vi "MecaDrivePoseEst_New.vi"(5 "gyroAngle":T5={"VALUE"=0.0, "COS"=1.0, "SIN"=0.0} {"SIN" format="%13.4f"; "COS" format="%13.4f"; "VALUE" format="%13.4f"}, 6 "MecanumKinematics":T1={"FrontLeft"={"X"=0.0, "Y"=0.0}, "FrontRight"={"X"=0.0, "Y"=0.0}, "RearLeft"={"X"=0.0, "Y"=0.0}, "RearRight"={"X"=0.0, "Y"=0.0}, "InverseKinematics"=[[0.0, 1.0, -1.0, 0.0], [0.0, 1.0, 1.0, 0.0], [0.0, 1.0, 1.0, 0.0], [0.0, 1.0, -1.0, 0.0]], "ForwardKinematics"=[[0.0, 1.0, -1.0, 0.0], [0.0, 1.0, 1.0, 0.0], [0.0, 1.0, 1.0, 0.0], [0.0, 1.0, -1.0, 0.0]], "PrevCoR"={"X"=0.0, "Y"=0.0}} {"PrevCoR"."Y" format="%14.3f"; "PrevCoR"."X" format="%14.3f"; "RearRight"."Y" format="%14.3f"; "RearRight"."X" format="%14.3f"; "RearLeft"."Y" format="%14.3f"; "RearLeft"."X" format="%14.3f"; "FrontRight"."Y" format="%14.3f"; "FrontRight"."X" format="%14.3f"; "FrontLeft"."Y" format="%14.3f"; "FrontLeft"."X" format="%14.3f"}, 7 "InitialPose":T4={"TRANSLATION"={"X"=0.0, "Y"=0.0}, "ROTATION"={"VALUE"=0.0, "COS"=1.0, "SIN"=0.0}} {"ROTATION"."SIN" format="%13.4f"; "ROTATION"."COS" format="%13.4f"; "ROTATION"."VALUE" format="%13.4f"; "TRANSLATION"."Y" format="%14.3f"; "TRANSLATION"."X" format="%14.3f"}, 8 "dt_Seconds":dbl=0.02, 9 "VisionMeasurementStdDevs":T3=[[0.0], [0.0], [0.0]], 10 "LocalMeasurementStdDevs":T3=[[0.0]], 11 "StateStdDevs":T3=[[0.0], [0.0], [0.0]]) -> (0 "Error":errorcluster, 3 "MecaDrivePoseEstimate":T6={"M_VisionContR"=[], "m_nominal_dT"=0.0, "m_PrevTime_Sec"=0.0, "m_GyroOffset"={"VALUE"=0.0, "COS"=1.0, "SIN"=0.0}, "m_PrevAngle"={"VALUE"=0.0, "COS"=1.0, "SIN"=0.0}, "m_Observer"={"m_P"=[], "m_xHat"=[], "States"=0, "Outputs"=0, "m_ContR"=[], "m_ContQ"=[], "m_SigmasF"=[], "m_dT_Sec"=0.0, "MERWE_SCALED_SIGMA_PTS"={"m_Wm"=[], "States"=0, "Alpha"=0.0, "m_Wc"=[], "Kappa"=0}, "meanFuncX"=refnum, "meanFuncY"=refnum, "residualFuncX"=refnum, "residualFuncY"=refnum, "addFuncX"=refnum, "addFuncXExtra"=variant, "residualFuncYExtra"=variant, "residualFuncXExtra"=variant, "MeanFuncYExtra"=variant, "MeanFuncXExtra"=variant, "Inputs"=0}, "m_kinematics"={"FrontLeft"={"X"=0.0, "Y"=0.0}, "FrontRight"={"X"=0.0, "Y"=0.0}, "RearLeft"={"X"=0.0, "Y"=0.0}, "RearRight"={"X"=0.0, "Y"=0.0}, "InverseKinematics"=[[0.0, 1.0, -1.0, 0.0], [0.0, 1.0, 1.0, 0.0], [0.0, 1.0, 1.0, 0.0], [0.0, 1.0, -1.0, 0.0]], "ForwardKinematics"=[[0.0, 1.0, -1.0, 0.0], [0.0, 1.0, 1.0, 0.0], [0.0, 1.0, 1.0, 0.0], [0.0, 1.0, -1.0, 0.0]], "PrevCoR"={"X"=0.0, "Y"=0.0}}, "Pose_Buffer"={"TimeStamps"=[], "Pose"=[], "Min_TimeStamp"=0.0, "Max_TimeStamp"=0.0, "ItemCount"=0, "MaxBufferTime"=0.0}} {"Pose_Buffer"."Pose"."ROTATION"."SIN" format="%13.4f"; "Pose_Buffer"."Pose"."ROTATION"."COS" format="%13.4f"; "Pose_Buffer"."Pose"."ROTATION"."VALUE" format="%13.4f"; "Pose_Buffer"."Pose"."TRANSLATION"."Y" format="%14.3f"; "Pose_Buffer"."Pose"."TRANSLATION"."X" format="%14.3f"; "m_kinematics"."PrevCoR"."Y" format="%14.3f"; "m_kinematics"."PrevCoR"."X" format="%14.3f"; "m_kinematics"."RearRight"."Y" format="%14.3f"; "m_kinematics"."RearRight"."X" format="%14.3f"; "m_kinematics"."RearLeft"."Y" format="%14.3f"; "m_kinematics"."RearLeft"."X" format="%14.3f"; "m_kinematics"."FrontRight"."Y" format="%14.3f"; "m_kinematics"."FrontRight"."X" format="%14.3f"; "m_kinematics"."FrontLeft"."Y" format="%14.3f"; "m_kinematics"."FrontLeft"."X" format="%14.3f"; "m_PrevAngle"."SIN" format="%13.4f"; "m_PrevAngle"."COS" format="%13.4f"; "m_PrevAngle"."VALUE" format="%13.4f"; "m_GyroOffset"."SIN" format="%13.4f"; "m_GyroOffset"."COS" format="%13.4f"; "m_GyroOffset"."VALUE" format="%13.4f"})   [LabVIEW 2019, in "Trajectory_Library.lvlib"]
doc: "Constructs a SwerveDrivePoseEstimator.\n\nThis class wraps an UnscentedKalmanFilter Unscented Kalman Filter to fuse latency-compensated vision measurements with swerve drive encoder velocity measurements. It will correct for noisy measurements and encoder drift. It is intended to be an easy but more accurate drop-in for SwerveDriveOdometry.\n \nSwerveDrivePoseEstimator_update should be called every robot loop. If your loops are faster or slower than the default of 0.02s, then you should change the nominal delta time using the calling parameter. \n \nSwerveDrivePoseEstimator_addVisionMeasurement can be called as infrequently as you want; if you never call it, then this class will behave mostly like regular encoder odometry.\n \nThe state-space system used internally has the following states (x), inputs (u), and outputs\n(y):\n \n x = [x, y, theta]? \n in the field coordinate system containing x position, \n y position, and heading.\n \n u = [v_l, v_r, dtheta]? \n containing left wheel velocity, right wheel velocity, \n and change in gyro heading.\n \n y = [x, y, theta]?\n from vision containing x position, y position, and\n heading; or <strong> y = [theta]? </strong> containing \n gyro heading.\n \n \nInputs:\n - gyroAngle -- The current gyro angle.\n - initialPoseMeters -- The starting pose estimate.\n - stateStdDevs -- Standard deviations of model states. Increase these numbers \n to trust your model's state estimates less. This matrix is in the form \n [x, y, theta]?, with units in meters and radians.\n - localMeasurementStdDevs -- Standard deviations of the encoder and gyro \n measurements. Increase these numbers to trust sensor readings from encoders \n and gyros less. This matrix is in the form [theta], with units in radians.\n - visionMeasurementStdDevs -- Standard deviations of the vision measurements. \n Increase these numbers to trust global measurements from vision less. \n This matrix is in the form [x, y,theta]?, with units in meters and radians.\n - nominalDtSeconds -- The time in seconds between each robot loop.\n - SwerveKinematics -- A correctly-configured kinematics object for your drivetrain.\n\n\nOutputs:\n - outSwevePoseEst -- Updated data cluster \n - Error -- If TRUE, an error occured."
uses:
  Trajectory_Library.lvlib
  MECA_DRIVE_POSE_EST.ctl
  <vilib>/Analysis/Matrix/Datatypes/RealMatrix.ctl
  ROTATION2D.ctl
  UNSCENTED_KALMAN_FILTER.ctl
  MERWE_SCALED_SIGMA_PTS.ctl
  CALLBACK_FUNC_TYPE.ctl
  MECA_DRIVE_KINEMATICS.ctl
  TRANSLATION2D.ctl
  TIME_INTERPOLATABLE_POSE.ctl
  POSE2D.ctl
  MatBuilder_Create.vi
  VecBuilder_3x1Fill.vi
  Pose2d_getXYAngle.vi
  Rotation2d_UnaryMinus.vi
  Rotation2d_RotateBy.vi
  Rotation2d_CreateAngle.vi
  Rotation2d_CreateXY.vi
  Util_CalcDist.vi
  <vilib>/Analysis/Matrix/NI_Matrix.lvlib
panel:
  in  "RightDistance_M":dbl
  in  "LeftDistance_M":dbl
  # "<3,1>"
  # "<1, 1>"
  # "<3, 1>"
  # "<3, 3>"
  # "State Estimate <Statess,1>"
  # "<States, States>"
  # "<States, ?>"
  # "<Statess,  States>"
  # "<Outputs, Outputs>"
  # "<?, 1>"
  # "<?, 1>"
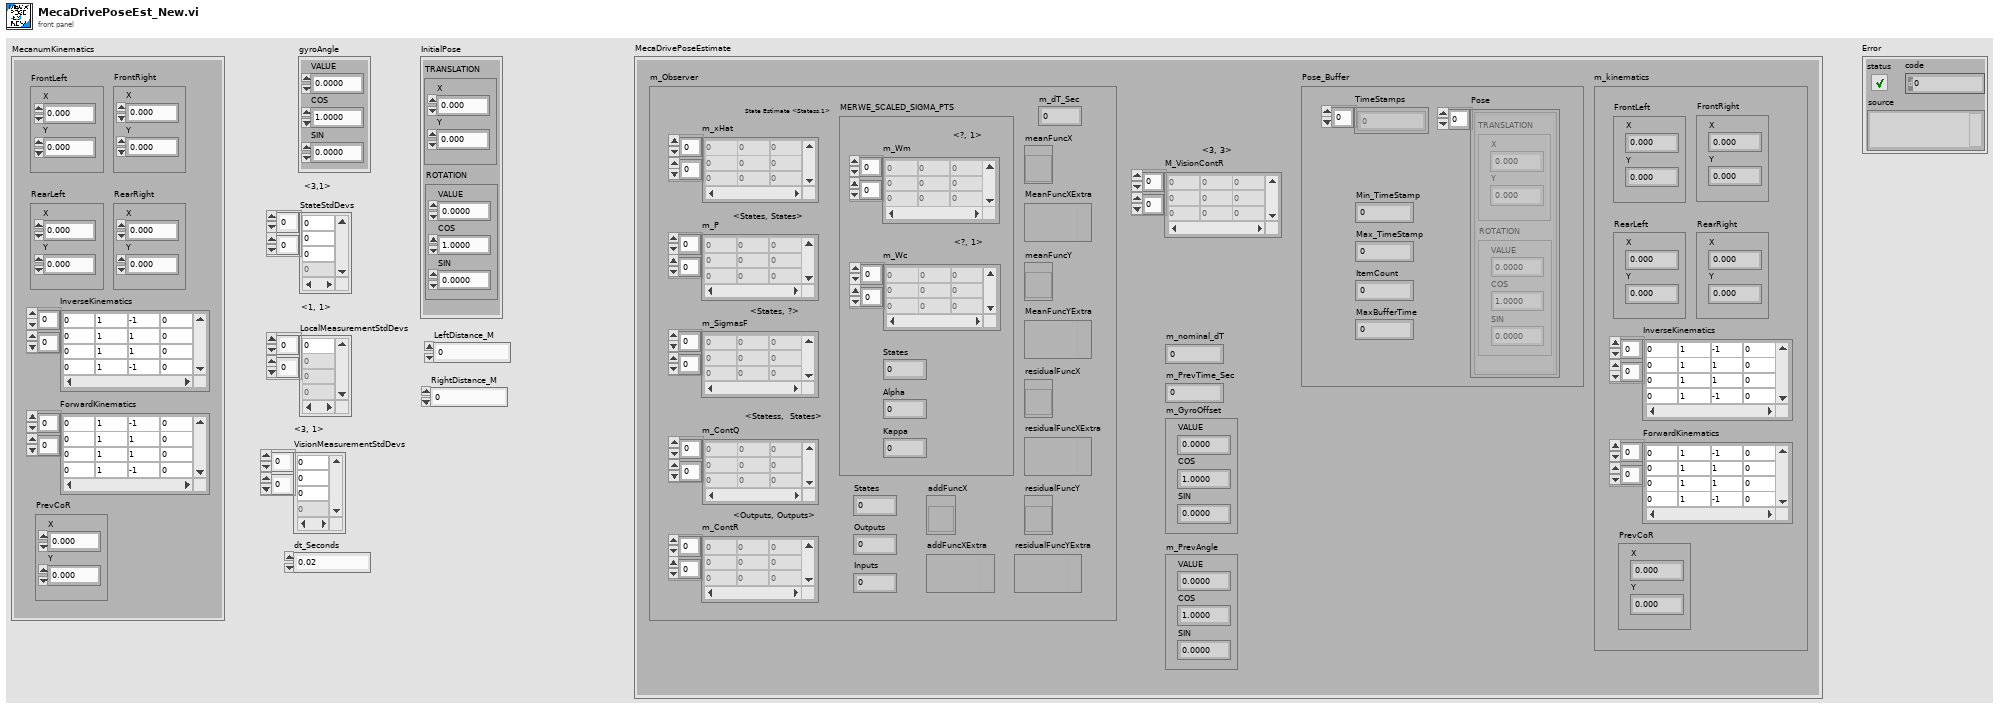
[diagram p1: front panel]
types:
  T1 = typedef "Trajectory_Library.lvlib/MECA_DRIVE_KINEMATICS.ctl" = cluster{"FrontLeft":T2, "FrontRight":T2, "RearLeft":T2, "RearRight":T2, "InverseKinematics":T3, "ForwardKinematics":T3, "PrevCoR":T2}
  T2 = typedef "Trajectory_Library.lvlib/TRANSLATION2D.ctl" = cluster{"X":dbl, "Y":dbl}
  T3 = typedef "NI_Matrix.lvlib/RealMatrix.ctl" = dbl[][]
  T4 = typedef "Trajectory_Library.lvlib/POSE2D.ctl" = cluster{"TRANSLATION":T2, "ROTATION":T5}
  T5 = typedef "Trajectory_Library.lvlib/ROTATION2D.ctl" = cluster{"VALUE":dbl, "COS":dbl, "SIN":dbl}
  T6 = typedef "Trajectory_Library.lvlib/MECA_DRIVE_POSE_EST.ctl" = cluster{"M_VisionContR":T3, "m_nominal_dT":dbl, "m_PrevTime_Sec":dbl, "m_GyroOffset":T5, "m_PrevAngle":T5, "m_Observer":T7, "m_kinematics":T1, "Pose_Buffer":T10}
  T7 = typedef "Trajectory_Library.lvlib/UNSCENTED_KALMAN_FILTER.ctl" = cluster{"m_P":T3, "m_xHat":T3, "States":i32, "Outputs":i32, "m_ContR":T3, "m_ContQ":T3, "m_SigmasF":T3, "m_dT_Sec":dbl, "MERWE_SCALED_SIGMA_PTS":T8, "meanFuncX":T9, "meanFuncY":T9, "residualFuncX":T9, "residualFuncY":T9, "addFuncX":T9, "addFuncXExtra":variant, "residualFuncYExtra":variant, "residualFuncXExtra":variant, "MeanFuncYExtra":variant, "MeanFuncXExtra":variant, "Inputs":i32}
  T8 = typedef "Trajectory_Library.lvlib/MERWE_SCALED_SIGMA_PTS.ctl" = cluster{"m_Wm":T3, "States":i32, "Alpha":dbl, "m_Wc":T3, "Kappa":i32}
  T9 = typedef "Trajectory_Library.lvlib/CALLBACK_FUNC_TYPE.ctl" = refnum<vi>
  T10 = typedef "Trajectory_Library.lvlib/TIME_INTERPOLATABLE_POSE.ctl" = cluster{"TimeStamps":dbl[], "Pose":T4[], "Min_TimeStamp":dbl, "Max_TimeStamp":dbl, "ItemCount":i32, "MaxBufferTime":dbl}
  T11 = typedef "Trajectory_Library.lvlib/UNSCENTED_KALMAN_NEW_FUNC_GROUP.ctl" = cluster{"meanFuncX":T9, "meanFuncY":T9, "residualFuncX":T9, "residualFuncY":T9, "addFuncX":T9, "MeanFuncXExtra":variant, "MeanFuncYExtra":variant, "residualFuncXExtra":variant, "residualFuncYExtra":variant, "addFuncXExtra":variant}
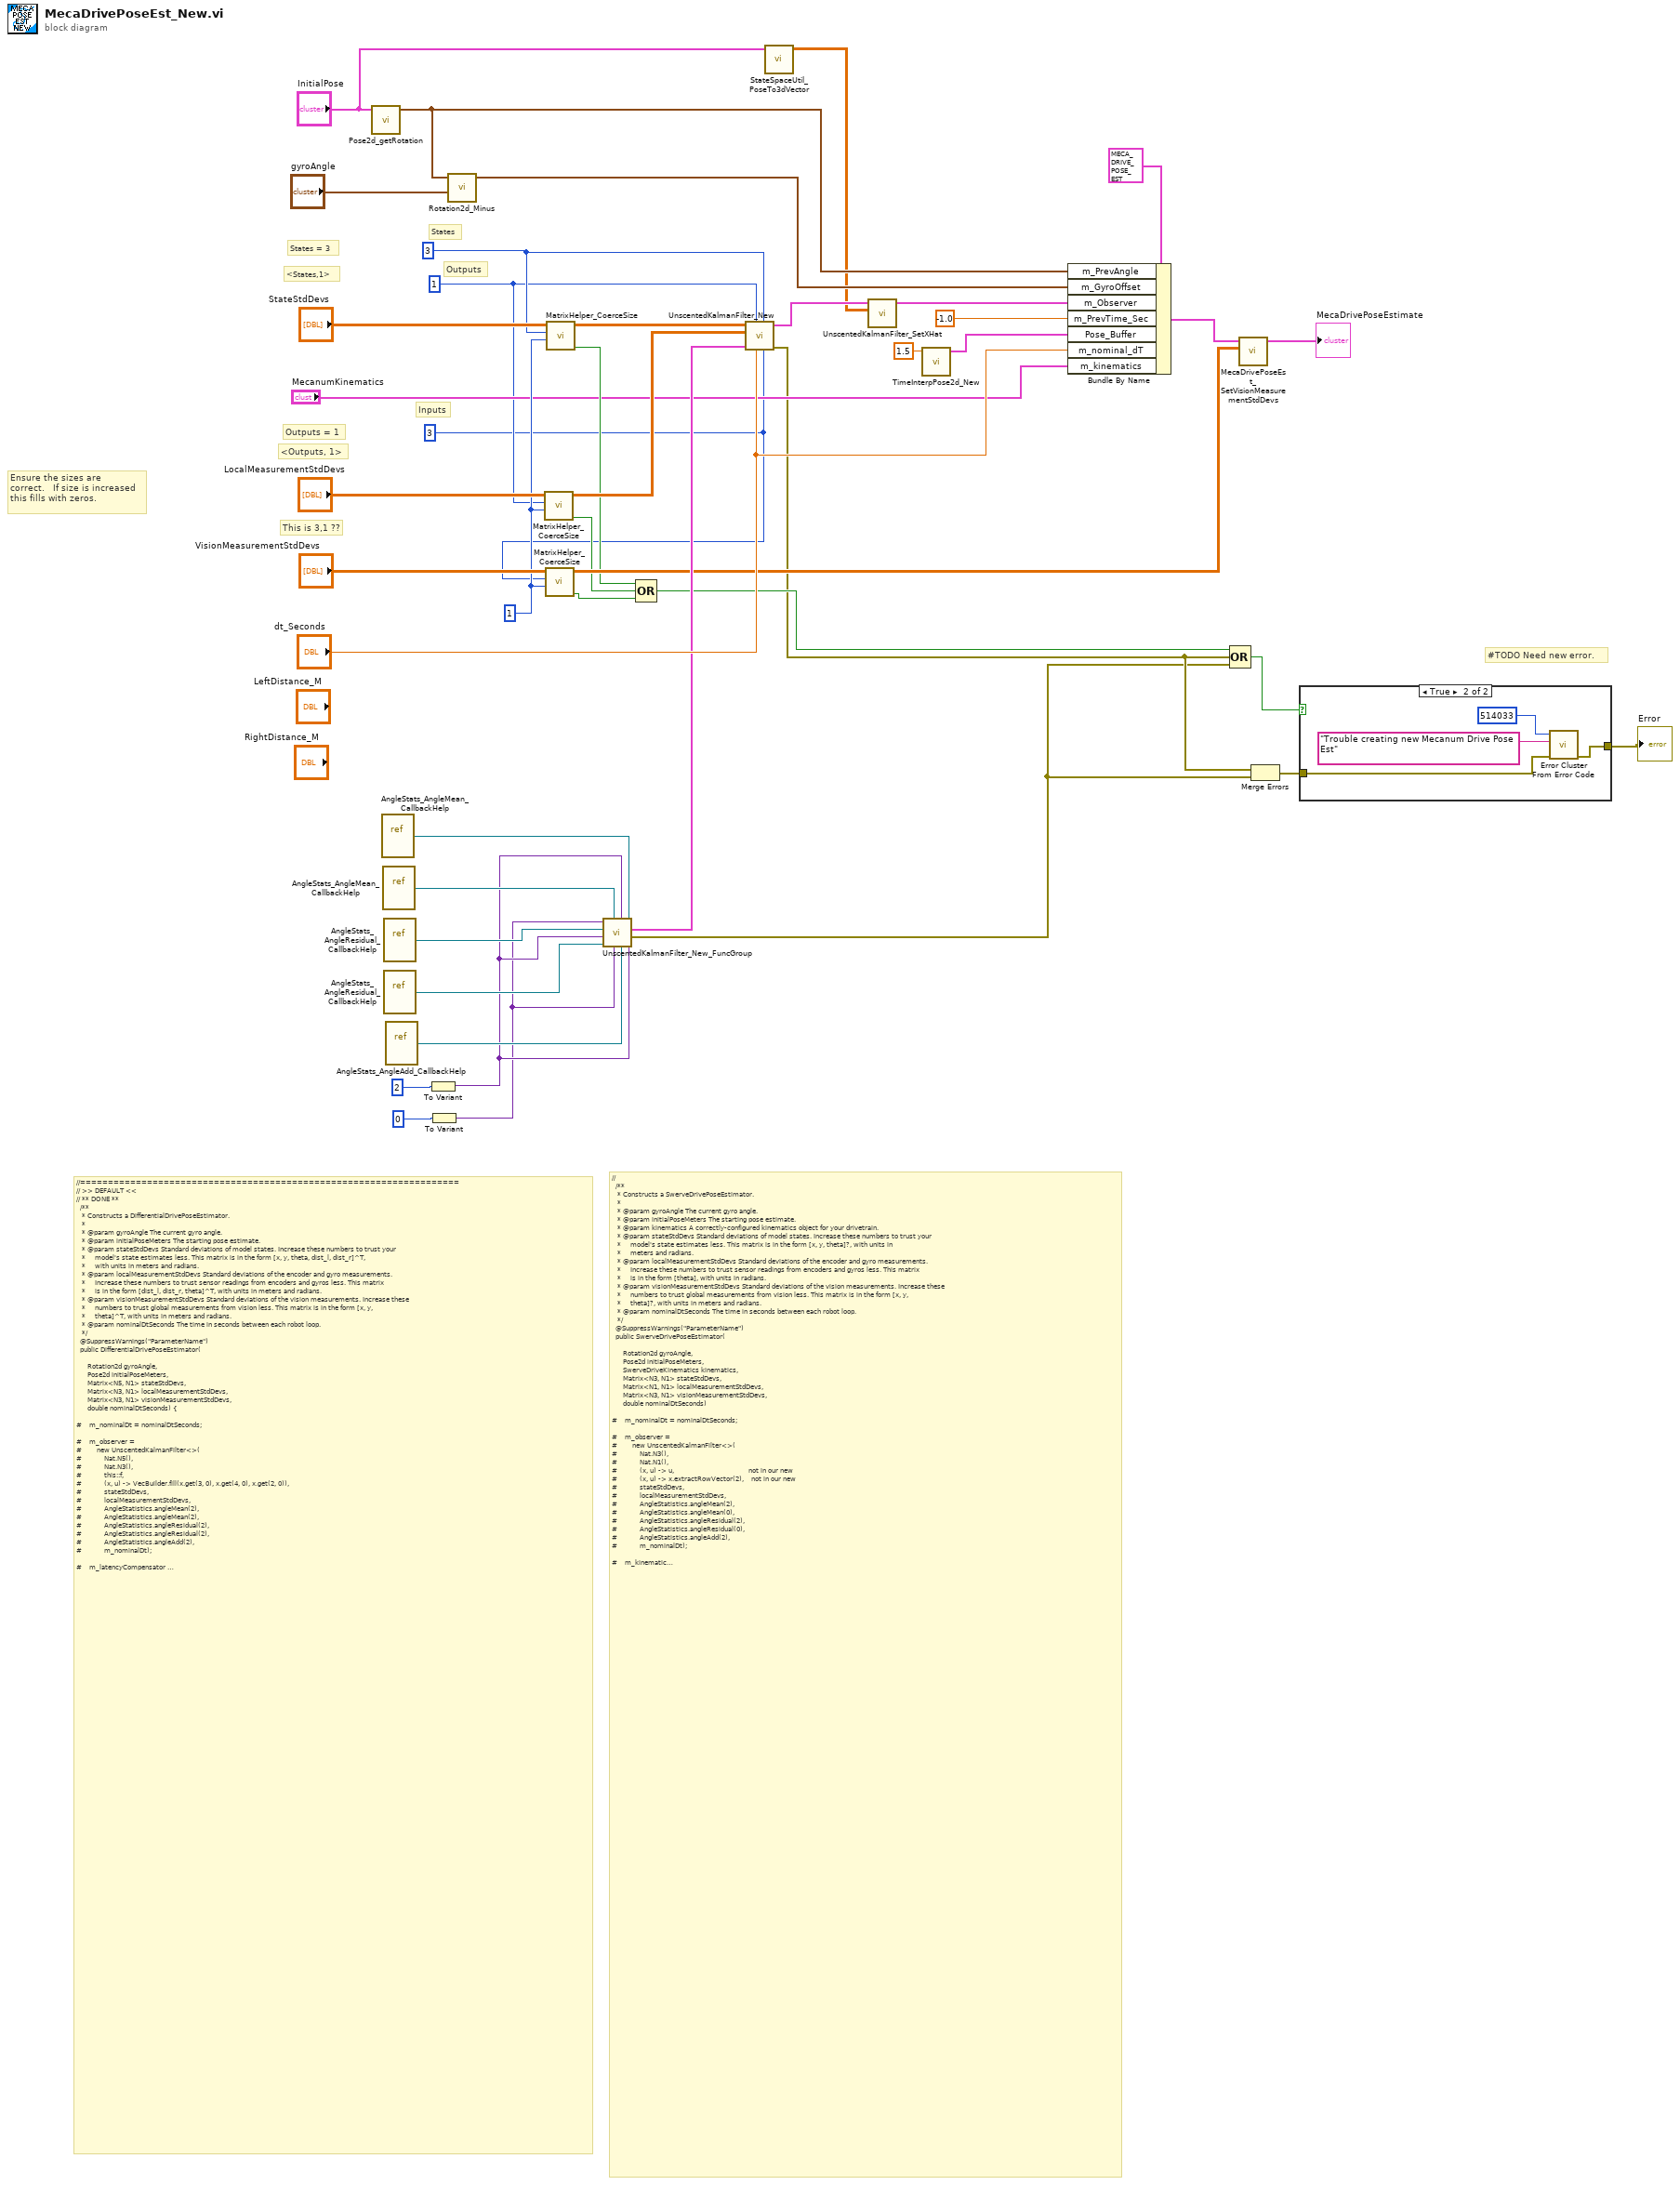
[diagram p0: block diagram]
diagram:
  w20 = 1 ("y")
  w10 = 3 ("Inputs")
  w11 = 1 ("Outputs")
  w19 = 3 ("States")
  # "#TODO Need new error."
  # "This is 3,1 ??"
  # "//====================================================================\n// >> DEFAULT <<\n// ** DONE **\n  /**\n   * Constructs a DifferentialDrivePoseEstimator.\n   *\n   * @param gyroAngle The current gyro angle.\n   * @param initialPoseMeters The starting pose estimate.\n   * @param stateStdDevs Standard deviations of model states. Increase these numbers to trust your\n   *     model's state estimates less. This matrix is in the form [x, y, theta, dist_l, dist_r]^T,\n   *     with units in meters and radians.\n   * @param localMeasurementStdDevs Standard deviations of the encoder and gyro measurements.\n   *     Increase these numbers to trust sensor readings from encoders and gyros less. This matrix\n   *     is in the form [dist_l, dist_r, theta]^T, with units in meters and radians.\n   * @param visionMeasurementStdDevs Standard deviations of the vision measurements. Increase these\n   *     numbers to trust global measurements from vision less. This matrix is in the form [x, y,\n   *     theta]^T, with units in meters and radians.\n   * @param nominalDtSeconds The time in seconds between each robot loop.\n   */\n  @SuppressWarnings(\"ParameterName\")\n  public DifferentialDrivePoseEstimator(\n\n      Rotation2d gyroAngle,\n      Pose2d initialPoseMeters,\n      Matrix<N5, N1> stateStdDevs,\n      Matrix<N3, N1> localMeasurementStdDevs,\n      Matrix<N3, N1> visionMeasurementStdDevs,\n      double nominalDtSeconds) {\n\n#    m_nominalDt = nominalDtSeconds;\n\n#    m_observer =\n#        new UnscentedKalmanFilter<>(\n#            Nat.N5(),\n#            Nat.N3(),\n#            this::f,\n#            (x, u) -> VecBuilder.fill(x.get(3, 0), x.get(4, 0), x.get(2, 0)),\n#            stateStdDevs,\n#            localMeasurementStdDevs,\n#            AngleStatistics.angleMean(2),\n#            AngleStatistics.angleMean(2),\n#            AngleStatistics.angleResidual(2),\n#            AngleStatistics.angleResidual(2),\n#            AngleStatistics.angleAdd(2),\n#            m_nominalDt);\n\n#    m_latencyCompensator = new KalmanFilterLatencyCompensator<>();\n\n#    // Initialize vision R\n#    setVisionMeasurementStdDevs(visionMeasurementStdDevs);\n\n//JAS not part of the data structure....\n    m_visionCorrect =\n        (u, y) ->\n            m_observer.correct(\n                Nat.N3(),\n                u,\n                y,\n                (x, u1) -> new Matrix<>(x.getStorage().extractMatrix(0, 3, 0, 1)),\n                m_visionDiscreteR,\n                AngleStatistics.angleMean(2),\n                AngleStatistics.angleResidual(2),\n                AngleStatistics.angleResidual(2),\n                AngleStatistics.angleAdd(2));\n\n#    m_gyroOffset = initialPoseMeters.getRotation().minus(gyroAngle);\n#    m_previousAngle = initialPoseMeters.getRotation();\n#    m_observer.setXhat(fillStateVector(initialPoseMeters, 0.0, 0.0));\n  }"
  # "// \n  /**\n   * Constructs a SwerveDrivePoseEstimator.\n   *\n   * @param gyroAngle The current gyro angle.\n   * @param initialPoseMeters The starting pose estimate.\n   * @param kinematics A correctly-configured kinematics object for your drivetrain.\n   * @param stateStdDevs Standard deviations of model states. Increase these numbers to trust your\n   *     model's state estimates less. This matrix is in the form [x, y, theta]?, with units in\n   *     meters and radians.\n   * @param localMeasurementStdDevs Standard deviations of the encoder and gyro measurements.\n   *     Increase these numbers to trust sensor readings from encoders and gyros less. This matrix\n   *     is in the form [theta], with units in radians.\n   * @param visionMeasurementStdDevs Standard deviations of the vision measurements. Increase these\n   *     numbers to trust global measurements from vision less. This matrix is in the form [x, y,\n   *     theta]?, with units in meters and radians.\n   * @param nominalDtSeconds The time in seconds between each robot loop.\n   */\n  @SuppressWarnings(\"ParameterName\")\n  public SwerveDrivePoseEstimator(\n\n      Rotation2d gyroAngle,\n      Pose2d initialPoseMeters,\n      SwerveDriveKinematics kinematics,\n      Matrix<N3, N1> stateStdDevs,\n      Matrix<N1, N1> localMeasurementStdDevs,\n      Matrix<N3, N1> visionMeasurementStdDevs,\n      double nominalDtSeconds) \n\n#    m_nominalDt = nominalDtSeconds;\n\n#    m_observer =\n#        new UnscentedKalmanFilter<>(\n#            Nat.N3(),\n#            Nat.N1(),\n#            (x, u) -> u,                                        not in our new\n#            (x, u) -> x.extractRowVector(2),    not in our new\n#            stateStdDevs,\n#            localMeasurementStdDevs,\n#            AngleStatistics.angleMean(2),\n#            AngleStatistics.angleMean(0),\n#            AngleStatistics.angleResidual(2),\n#            AngleStatistics.angleResidual(0),\n#            AngleStatistics.angleAdd(2),\n#            m_nominalDt);\n\n#    m_kinematics = kinematics;\n\n#    m_latencyCompensator = new KalmanFilterLatencyCompensator<>();\n\n#    // Initialize vision R\n#    setVisionMeasurementStdDevs(visionMeasurementStdDevs);\n\n//JAS not part of the data structure....\n    m_visionCorrect =\n        (u, y) ->\n            m_observer.correct(\n                Nat.N3(),\n                u,\n                y,\n                (x, u1) -> x,\n                m_visionContR,\n                AngleStatistics.angleMean(2),\n                AngleStatistics.angleResidual(2),\n                AngleStatistics.angleResidual(2),\n                AngleStatistics.angleAdd(2));\n\n#    m_gyroOffset = initialPoseMeters.getRotation().minus(gyroAngle);\n#    m_previousAngle = initialPoseMeters.getRotation();\n#    m_observer.setXhat(  StateSpaceUtil.poseTo3dVector(initialPoseMeters));\n  }"
  # "Inputs"
  # "Outputs = 1"
  # "States = 3"
  # "Outputs"
  # "States"
  # "<Outputs, 1>"
  # "<States,1>"
  # "Ensure the sizes are\ncorrect.   If size is increased \nthis fills with zeros."
  n1 = call "Pose2d_getRotation.vi"("in POSE"="InitialPose") -> ("out ROTATION"=w40:T5)  [unwired: 10 in]
  n2 = vi-ref "AngleStats_AngleMean_CallbackHelp.vi"() -> (w33:refnum<vi>)
  n3 = vi-ref "AngleStats_AngleMean_CallbackHelp.vi"() -> (w32:refnum<vi>)
  n4 = vi-ref "AngleStats_AngleResidual_CallbackHelp.vi"() -> (w31:refnum<vi>)
  n5 = vi-ref "AngleStats_AngleResidual_CallbackHelp.vi"() -> (w30:refnum<vi>)
  n6 = vi-ref "AngleStats_AngleAdd_CallbackHelp.vi"() -> (w28:refnum<vi>)
  n7 = To Variant(anything=2) -> (Variant=w27:variant)
  n8 = To Variant(anything=0) -> (Variant=w13:variant)
  n9 = call "Rotation2d_Minus.vi"("other ROTATION"="gyroAngle", "in ROTATION"=w40) -> ("out ROTATION"=w41:T5)  [unwired: 9 in]
  n10 = call "MatrixHelper_CoerceSize.vi"("Columns"=w20, "Rows"=w11, "input matrix"="LocalMeasurementStdDevs") -> ("Coerced"=w16:bool, "output matrix"=w25:T3)  [unwired: 7 in]
  n11 = call "MatrixHelper_CoerceSize.vi"("Columns"=w20, "Rows"=w10, "input matrix"="VisionMeasurementStdDevs") -> ("Coerced"=w15:bool, "output matrix"=w21:T3)  [unwired: 7 in]
  n12 = call "MatrixHelper_CoerceSize.vi"("Columns"=w20, "Rows"=w19, "input matrix"="StateStdDevs") -> ("Coerced"=w17:bool, "output matrix"=w23:T3)  [unwired: 7 in]
  n13 = call "UnscentedKalmanFilter_New_FuncGroup.vi"("addFuncXExtra"=w27, "MeanFuncX"=w33, "AddFuncX"=w28, "MeanFuncXExtra"=w27, "residualFuncYExtra"=w13, "MeanFuncY"=w32, "ResidualFuncY"=w30, "residualFuncXExtra"=w27, "ResidualFuncX"=w31, "MeanFuncYExtra"=w13) -> ("Error"=w4:errorcluster, "UNSCENTED_KALMAN_NEW_FUNC_GROUP"=w34:T11)
  n14 = Compound Arithmetic op=OR(w17, w16, w15) -> (w18:bool)
  n15 = call "UnscentedKalmanFilter_New.vi"("Inputs"=w10, "States"=w19, "dt_Seconds"="dt_Seconds", "Outputs"=w11, "UNSCENTED_KALMAN_NEW_FUNC_GROUP"=w34, "MeasurementStdDevs"=w25, "StateStdDevs"=w23) -> ("Error"=w5:errorcluster, "UnscentedKalmanFiilter"=w38:T7)  [unwired: 3 in]
  n16 = call "StateSpaceUtil_PoseTo3dVector.vi"("Pose"="InitialPose") -> ("Pose Vector"=w9:T3)  [unwired: 10 in]
  n17 = call "UnscentedKalmanFilter_SetXHat.vi"("xHat"=w9, "in UnscentedKalmanFiilter"=w38) -> ("out UnscentedKalmanFiilter"=w39:T7)  [unwired: 8 in, 1 out]
  n18 = call "TimeInterpPose2d_New.vi"("MaxTime"=1.5) -> ("TimeInterpPose"=w1:T10)  [unwired: 10 in]
  n19 = Bundle By Name(cluster=T6 {"M_VisionContR"=[], "m_nominal_dT"=0.0, "m_PrevTime_Sec"=0.0, "m_GyroOffset"={"VALUE"=0.0, "COS"=1.0, "SIN"=0.0}, "m_PrevAngle"={"VALUE"=0.0, "COS"=1.0, "SIN"=0.0}, "m_Observer"={"m_P"=[], "m_xHat"=[], "States"=0, "Outputs"=0, "m_ContR"=[], "m_ContQ"=[], "m_SigmasF"=[], "m_dT_Sec"=0.0, "MERWE_SCALED_SIGMA_PTS"={"m_Wm"=[], "States"=0, "Alpha"=0.0, "m_Wc"=[], "Kappa"=0}, "meanFuncX"=refnum, "meanFuncY"=refnum, "residualFuncX"=refnum, "residualFuncY"=refnum, "addFuncX"=refnum, "addFuncXExtra"=variant, "residualFuncYExtra"=variant, "residualFuncXExtra"=variant, "MeanFuncYExtra"=variant, "MeanFuncXExtra"=variant, "Inputs"=0}, "m_kinematics"={"FrontLeft"={"X"=0.0, "Y"=0.0}, "FrontRight"={"X"=0.0, "Y"=0.0}, "RearLeft"={"X"=0.0, "Y"=0.0}, "RearRight"={"X"=0.0, "Y"=0.0}, "InverseKinematics"=[[0.0, 1.0, -1.0, 0.0], [0.0, 1.0, 1.0, 0.0], [0.0, 1.0, 1.0, 0.0], [0.0, 1.0, -1.0, 0.0]], "ForwardKinematics"=[[0.0, 1.0, -1.0, 0.0], [0.0, 1.0, 1.0, 0.0], [0.0, 1.0, 1.0, 0.0], [0.0, 1.0, -1.0, 0.0]], "PrevCoR"={"X"=0.0, "Y"=0.0}}, "Pose_Buffer"={"TimeStamps"=[], "Pose"=[], "Min_TimeStamp"=0.0, "Max_TimeStamp"=0.0, "ItemCount"=0, "MaxBufferTime"=0.0}} ("DIFF_DRIVE_POSE_EST"), "m_PrevAngle"=w40, "m_GyroOffset"=w41, "m_Observer"=w39, "m_PrevTime_Sec"=-1.0, "Pose_Buffer"=w1, "m_nominal_dT"="dt_Seconds", "m_kinematics"="MecanumKinematics") -> (w37:T6)
  n20 = Compound Arithmetic op=OR(w18, w5, w4) -> (w6:bool)
  n21 = call "MecaDrivePoseEst_SetVisionMeasurementStdDevs.vi"("VisionMeasurementStdDevs"=w21, "in MecaDrivePoseEstimate"=w37) -> ("Out MecaDrivePoseEstimate"=→"MecaDrivePoseEstimate":T6)  [unwired: 8 in, 1 out]
  n22 = Merge Errors(w5, w4) -> (w7:errorcluster)
  n23 = case shown="True" w6 {
    tunnel: w7 -> [w45 w48]
    tunnel: [w45 w49] -> w3
    frame False {
    }
    frame True {
      n24 = call <vilib>:"Error Cluster From Error Code.vi"("error in (no error)"=w48, "error message (\"\")"="Trouble creating new Mecanum Drive Pose Est" ("error message (\"\")"), "error code (0)"=514033) -> ("error out"=w49:errorcluster)  [unwired: 6 in]
    }
  }
  "Error" <- w3
